vi "Demo.vi"   [LabVIEW 2019]
uses:
  builds/KNRm_ReMi_Toolkit/KNRm/KNRm_ReMi_OS6/home/lvuser/natinst/bin/KNRm_ReMi_OS6.lvlibp
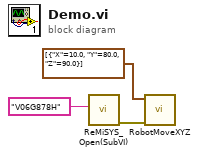
[diagram p0: block diagram]
diagram:
  n1 = call "ReMiSYS_Open(SubVI).vi"("ReMiSYS Key"="V06G878H") -> ("error out"=w2:errorcluster)  [unwired: 9 in, 1 out]
  n2 = call "RobotMoveXYZ.vi"("error in"=w2, "Movement [X,Y,Z] (cm,cm,deg)"=cluster{"X":dbl, "Y":dbl, "Z":dbl}[] [{"X"=10.0, "Y"=80.0, "Z"=90.0}]) -> ()  [unwired: 8 in, 2 out]
